vi "read_2ch_flexRIO.vi"(10 "channel offsets":T1) -> (2 "read output":T1)   [LabVIEW 2010]
uses:
  channels_cluster_flexRIO.ctl
  <vilib>/eio/EIONode/EIONode.xnode
  <vilib>/rvi/eio/nirviEIOImplementation/nirviEIOImplementation.xnode
  <vilib>/rvi/eio/common/nirviEmuClasses.ctl
  <vilib>/rvi/eio/common/nirviEmuTemplateMethod_noerrors.vi
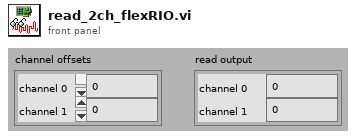
[diagram p1: front panel]
types:
  T1 = typedef "channels_cluster_flexRIO.ctl" = cluster{"channel 0":u32, "channel 1":u32}
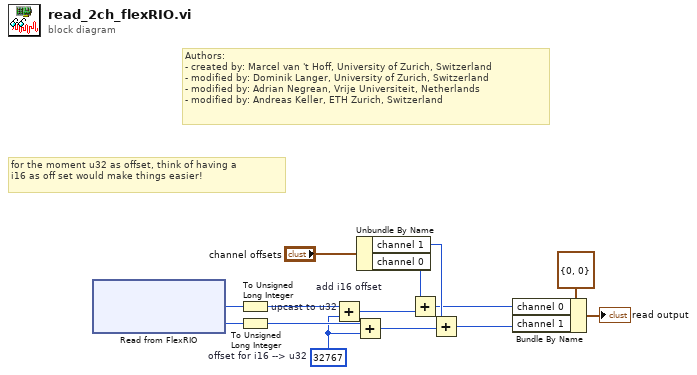
[diagram p0: block diagram]
diagram:
  w10 = u32 32767  # offset for i16 --> u32
  # "for the moment u32 as offset, think of having a\ni16 as off set would make things easier!"
  # "Authors: \n- created by: Marcel van 't Hoff, University of Zurich, Switzerland\n- modified by: Dominik Langer, University of Zurich, Switzerland\n- modified by: Adrian Negrean, Vrije Universiteit, Netherlands\n- modified by: Andreas Keller, ETH Zurich, Switzerland"
  n1 = xnode "Read from FlexRIO"() -> ("IO Module\\AI A0"=w13:i16, "IO Module\\AI A1"=w14:i16)  [unwired: 2 in, 2 out]
  n2 = To Unsigned Long Integer "upcast to u32"(number=w13) -> (unsigned 32bit integer=w12:u32)
  n3 = To Unsigned Long Integer(number=w14) -> (unsigned 32bit integer=w11:u32)
  n4 = Add "add i16 offset"(x=w12, y=w10) -> (x+y=w9:u32)
  n5 = Add(x=w11, y=w10) -> (x+y=w8:u32)
  n6 = Unbundle By Name("channel offsets") -> ("channel 1"=w7:u32, "channel 0"=w6:u32)
  n7 = Add(x=w6, y=w9) -> (x+y=w5:u32)
  n8 = Add(x=w7, y=w8) -> (x+y=w4:u32)
  n9 = Bundle By Name(cluster=T1 {"channel 0"=0, "channel 1"=0} ("read output"), "channel 0"=w5, "channel 1"=w4) -> (→"read output":T1)
